vi "log_subVI.vi"(0 "Path":path, 1 "Name":string="Name", 2 "Surname":string, 5 "True Value":string, 7 "Incremented":string, 9 "Error":string, 11 "Error In":errorcluster, 12 "Lab":string, 13 "Instrument":string) -> (15 "Error Out":errorcluster)   [LabVIEW 2021, in "Main.lvlib" / "Main_Programs_SubVIs.lvlib"]
doc: "This subVI is used to write the the data to csv or txt file."
uses:
  Main_Programs_SubVIs.lvlib
  <vilib>/Utility/config.llb/Write Key (String).vi
  <vilib>/Utility/file.llb/Read Delimited Spreadsheet (string).vi
  <vilib>/Utility/file.llb/Write Delimited Spreadsheet (string).vi
  <vilib>/Utility/config.llb/NI_LVConfig.lvlib
panel:
  # "Input"
  # "Output"
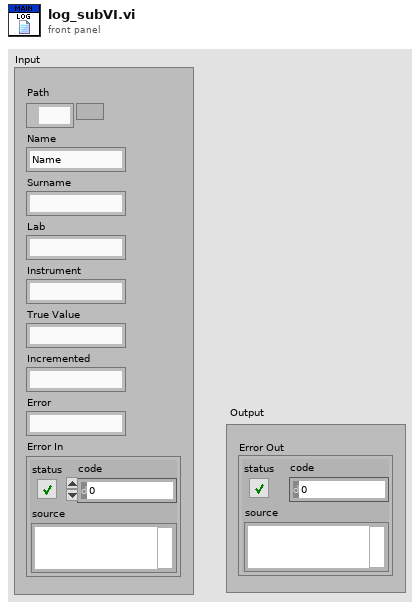
[diagram p1: front panel]
types:
  T1 = typedef "NI_LVConfig.lvlib/Config Data RefNum.ctl" = refnum<k1>
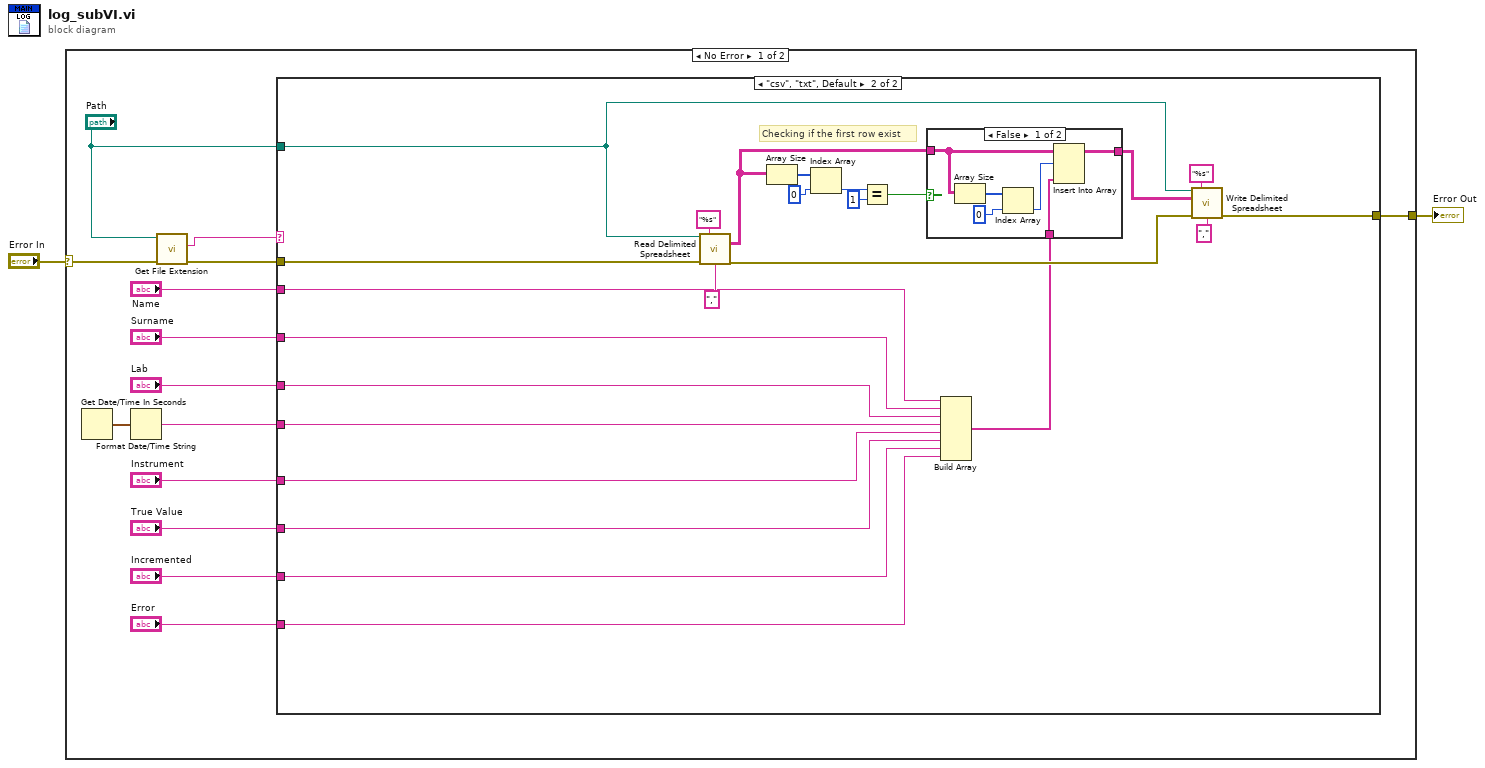
[diagram p0: block diagram]
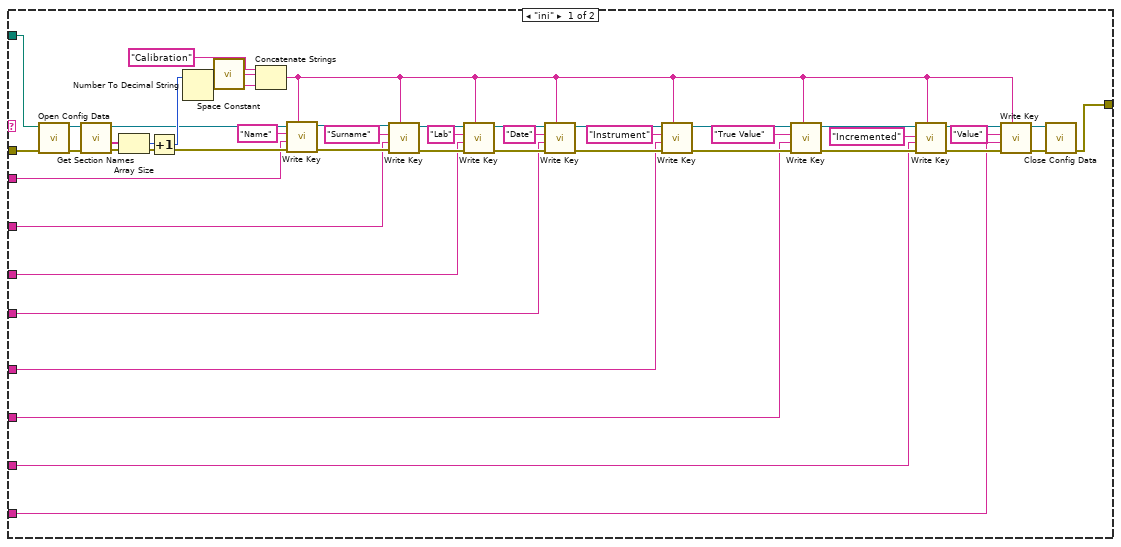
[diagram p2: hidden frame]
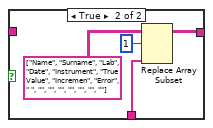
[diagram p3: hidden frame]
diagram:
  n1 = case shown="No Error" "Error In" {
    selector: "Error In" -> [w6 w97]
    tunnel: [w16 w97] -> w1
    frame No Error {
      n2 = Get Date/Time In Seconds() -> (seconds since 1Jan1904=w15:timestamp)
      n3 = Format Date/Time String(seconds (now)=w15) -> (date/time string=w9:string)  [unwired: 2 in]
      n4 = call <vilib>:"Get File Extension.vi"("error in (no error)"=w6, "file"="Path") -> ("error out"=w5:errorcluster, "lowercase file extension"=w3:string)  [unwired: 5 in, 3 out]
      n5 = case shown="\"csv\", \"txt\", Default" w3 {
        tunnel: w5 -> [w62 w84]
        tunnel: [w18 w80] -> w16
        tunnel: "Name" -> [w43 w79]
        tunnel: "Error" -> [w20 w78]
        tunnel: "Incremented" -> [w21 w77]
        tunnel: "True Value" -> [w27 w76]
        tunnel: "Instrument" -> [w33 w75]
        tunnel: w9 -> [w37 w74]
        tunnel: "Lab" -> [w41 w73]
        tunnel: "Surname" -> [w42 w72]
        tunnel: "Path" -> [w61 w71]
        frame "ini" {
          n6 = call <vilib>:"Open Config Data.vi"("error in (no error)"=w62, "configuration file path"=w61) -> ("error out"=w60:errorcluster, "refnum"=w59:T1)  [unwired: 7 in, 1 out]
          n7 = call <vilib>:"Get Section Names.vi"("error in (no error)"=w60, "refnum"=w59) -> ("error out"=w52:errorcluster, "section names"=w58:string[], "refnum out"=w51:T1)  [unwired: 7 in]
          n8 = Array Size(array=w58) -> (size(s)=w57:i32)
          n9 = Increment(x=w57) -> (x+1=w56:i32)
          n10 = Number To Decimal String(number=w56) -> (decimal integer string=w55:string)  [unwired: 1 in]
          n11 = call <vilib>:"Space Constant.vi"() -> ("String"=w53:string)
          n12 = Concatenate Strings("Calibration" ("string"), w53, w55) -> (w17:string)
          n13 = call-poly <vilib>:"Write Key.vi"("section"=w17, "error in (no error)"=w52, "value"=w43, "key"="Name", "refnum"=w51) -> ("error out"=w45:errorcluster, "refnum out"=w50:T1)  [unwired: 4 in, 1 out]
          n14 = call-poly <vilib>:"Write Key.vi"("section"=w17, "error in (no error)"=w45, "value"=w42, "key"="Surname", "refnum"=w50) -> ("error out"=w46:errorcluster, "refnum out"=w47:T1)  [unwired: 4 in, 1 out]
          n15 = call-poly <vilib>:"Write Key.vi"("section"=w17, "error in (no error)"=w46, "value"=w41, "key"="Lab", "refnum"=w47) -> ("error out"=w39:errorcluster, "refnum out"=w40:T1)  [unwired: 4 in, 1 out]
          n16 = call-poly <vilib>:"Write Key.vi"("section"=w17, "error in (no error)"=w39, "value"=w37, "key"="Date", "refnum"=w40) -> ("error out"=w36:errorcluster, "refnum out"=w35:T1)  [unwired: 4 in, 1 out]
          n17 = call-poly <vilib>:"Write Key.vi"("section"=w17, "error in (no error)"=w36, "value"=w33, "key"="Instrument", "refnum"=w35) -> ("error out"=w31:errorcluster, "refnum out"=w32:T1)  [unwired: 4 in, 1 out]
          n18 = call-poly <vilib>:"Write Key.vi"("section"=w17, "error in (no error)"=w31, "value"=w27, "key"="True Value", "refnum"=w32) -> ("error out"=w29:errorcluster, "refnum out"=w28:T1)  [unwired: 4 in, 1 out]
          n19 = call-poly <vilib>:"Write Key.vi"("section"=w17, "error in (no error)"=w29, "value"=w21, "key"="Incremented", "refnum"=w28) -> ("error out"=w24:errorcluster, "refnum out"=w25:T1)  [unwired: 4 in, 1 out]
          n20 = call-poly <vilib>:"Write Key.vi"("section"=w17, "error in (no error)"=w24, "value"=w20, "key"="Value", "refnum"=w25) -> ("error out"=w22:errorcluster, "refnum out"=w23:T1)  [unwired: 4 in, 1 out]
          n21 = call <vilib>:"Close Config Data.vi"("error in (no error)"=w22, "refnum"=w23) -> ("error out"=w18:errorcluster)  [unwired: 8 in, 1 out]
        }
        frame "csv", "txt", Default {
          # "Checking if the first row exist"
          n22 = call-poly <vilib>:"Read Delimited Spreadsheet.vi"("file path (dialog if empty)"=w71, "format (%s)"="%s", "error in (no error)"=w84, "delimiter (\\t)"="," ("delimiter (\\t)")) -> ("all rows"=w64:string[][], "error out"=w83:errorcluster)  [unwired: 6 in, 4 out]
          n23 = Array Size(array=w64) -> (size(s)=w69:i32[])
          n24 = Index Array(array=w69, index=0) -> (element=w70:i32)
          n25 = Equal?(x=w70, y=1) -> (x = y?=w66:bool)
          n26 = Build Array(w79, w72, w73, w74, w75, w76, w77, w78) -> (w65:string[])
          n27 = case shown="False" w66 {
            tunnel: w65 -> [w91 w93]
            tunnel: w64 -> [w89 _]
            tunnel: [w88 w96] -> w63
            frame False {
              n28 = Array Size(array=w89) -> (size(s)=w92:i32[])
              n29 = Index Array(array=w92, index=0) -> (element=w87:i32)
              n30 = Insert Into Array(array=w89, index (row)=w87, new element=w91) -> (w88:string[][])  [unwired: 1 in]
            }
            frame True {
              n31 = Replace Array Subset(array=string[][] [["Name", "Surname", "Lab", "Date", "Instrument", "True Value", "Incremen", "Error"], [" ", "", "", "", "", "", "", ""]], new element=w93, index (row)=1) -> (w96:string[][])  [unwired: 1 in]
            }
          }
          n32 = call-poly <vilib>:"Write Delimited Spreadsheet.vi"("file path (dialog if empty)"=w71, "format (%s)"="%s", "2D data"=w63, "error in (no error)"=w83, "delimiter (\\t)"="," ("delimiter (\\t)")) -> ("error out"=w80:errorcluster)  [unwired: 9 in, 1 out]
        }
      }
    }
    frame Error {
    }
  }
  "Error Out" <- w1
